vi "KIMTest.vi"() -> ()   [LabVIEW 2018, in "KIM101lib.lvlib"]
doc: "Use this template to build a producer/consumer design pattern with events to produce queue items. Use this design pattern instead of the User Interface Event Handler pattern for user interfaces when you want to execute code asynchronously in response to an event without slowing the user interface responsiveness."
uses:
  KIM101lib.lvlib
panel:
  in  "APTPZMotor":refnum<k7>(container)
  out "状态":i32[](array[numeric])
  in  "设置0位":bool
  in  "轴4":T1
  in  "轴3":T2
  in  "轴2":T3
  in  "轴1":T3
  out "Position":i32[](array[numeric])
  in  "stop":bool
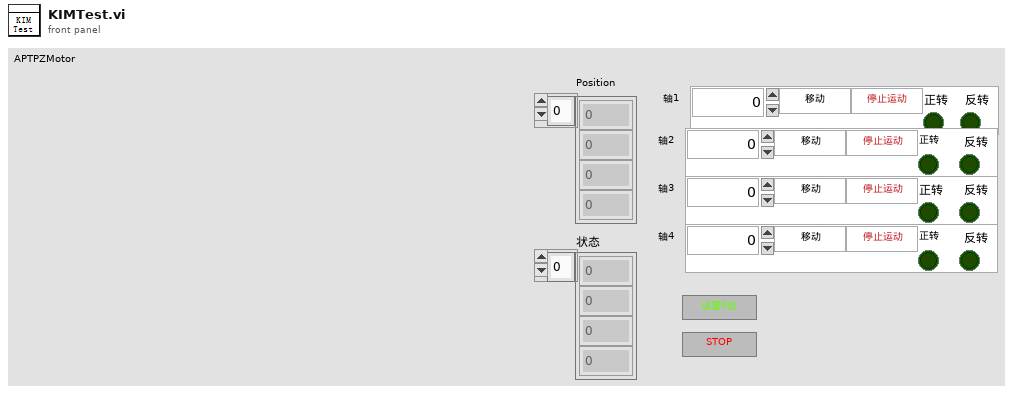
[diagram p1: front panel]
types:
  T1 = cluster{"目标位置":i32, "移动":bool, "停止运动":bool, "正转":bool, " 反转":bool}
  T2 = cluster{"目标位置":i32, "移动":bool, "停止运动":bool, "正转  ":bool, " 反转":bool}
  T3 = cluster{"目标位置":i32, "移动":bool, "停止运动":bool, "正转 ":bool, " 反转":bool}
  T4 = cluster{"电压(80-130)":i32, "速度(1-2000) ":i32, "加速度(1-100000)":i32}
  T5 = enum16{"全部禁用", "CH1使能", "CH2使能", "CH3使能", "CH4使能", "CH1,CH2使能", "CH3,CH4使能"}
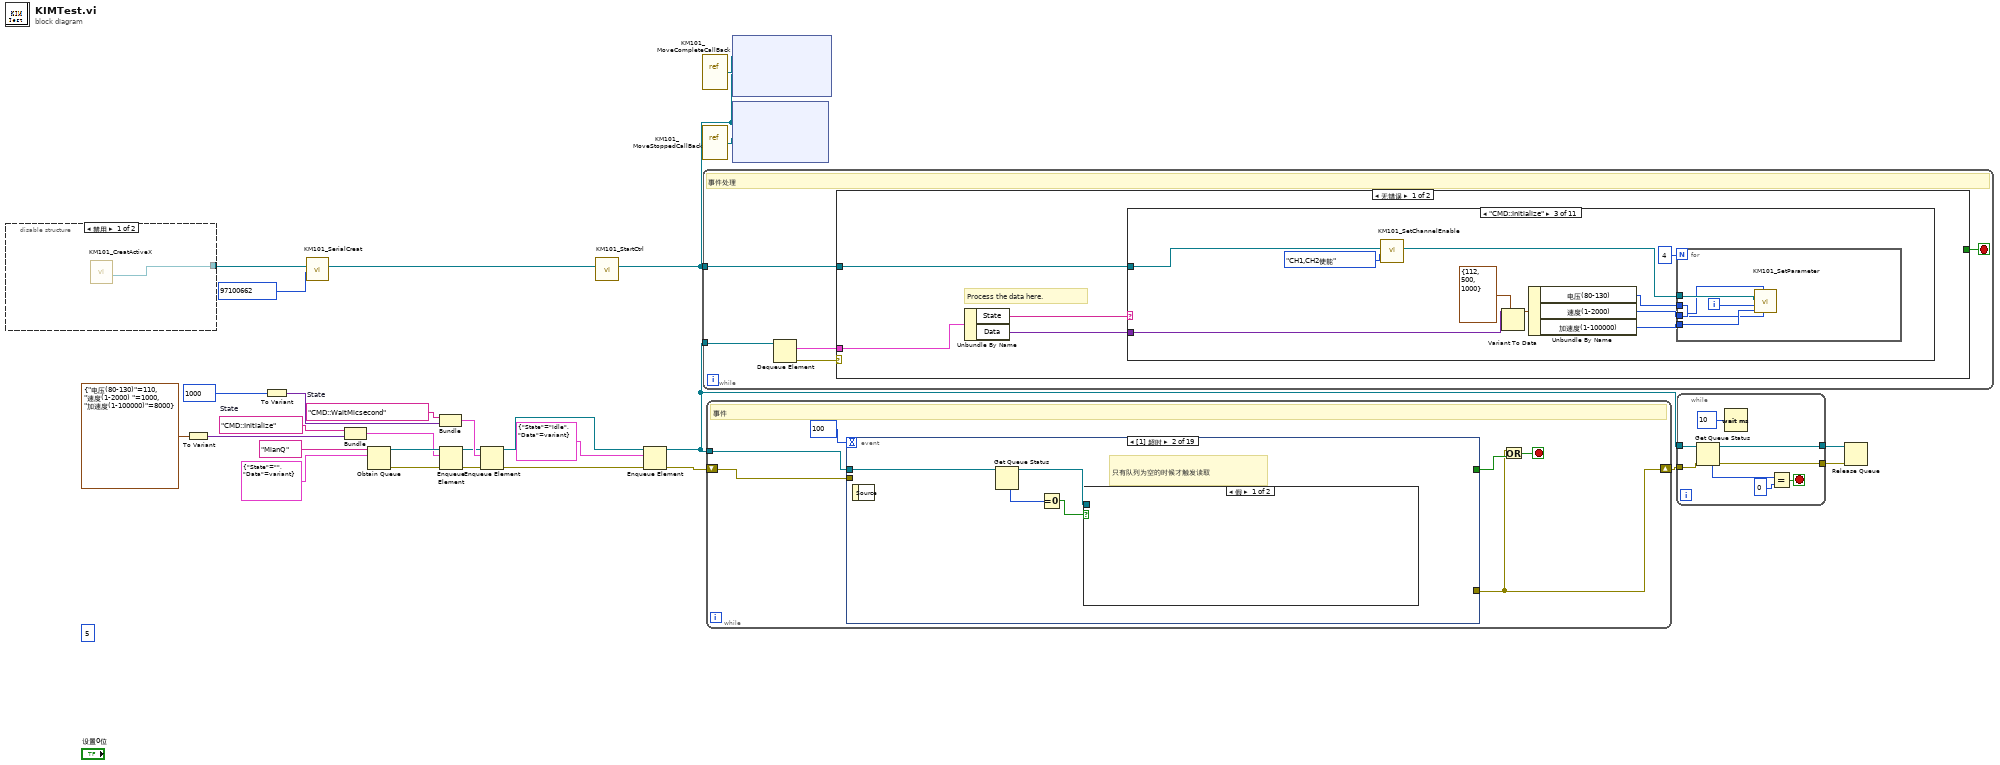
[diagram p0: block diagram]
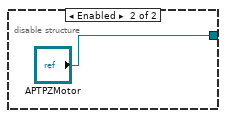
[diagram p2: hidden frame]
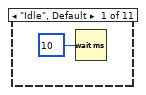
[diagram p3: hidden frame]
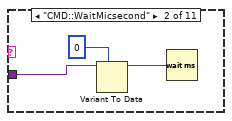
[diagram p4: hidden frame]
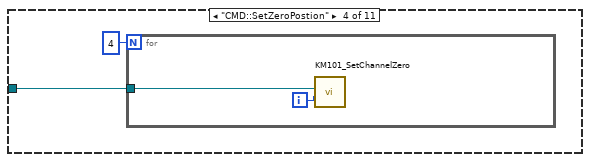
[diagram p5: hidden frame]
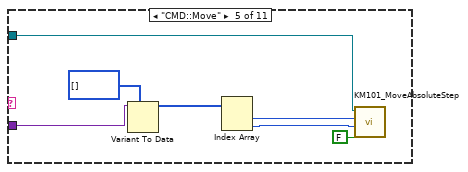
[diagram p6: hidden frame]
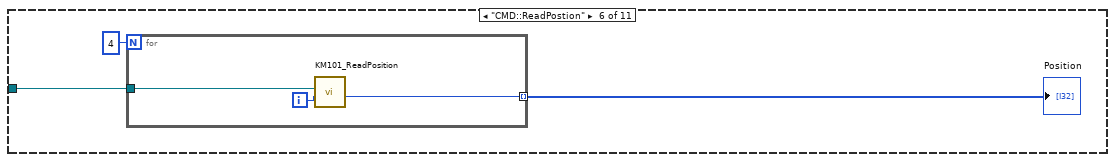
[diagram p7: hidden frame]
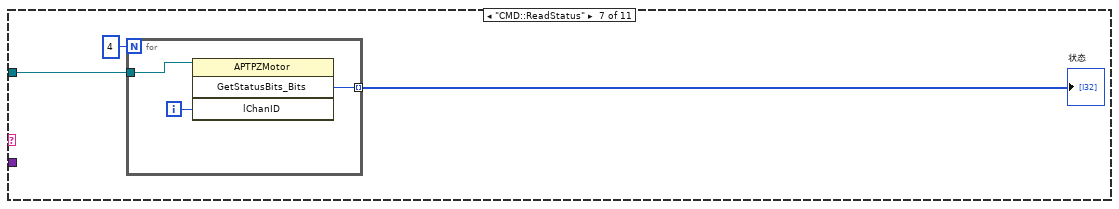
[diagram p8: hidden frame]
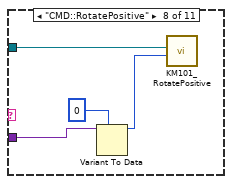
[diagram p9: hidden frame]
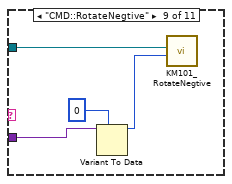
[diagram p10: hidden frame]
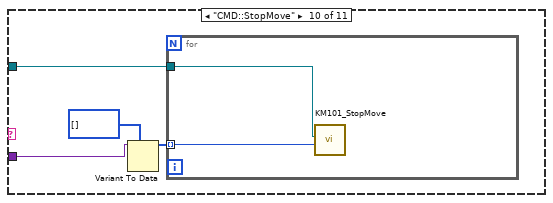
[diagram p11: hidden frame]
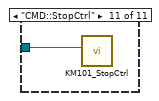
[diagram p12: hidden frame]
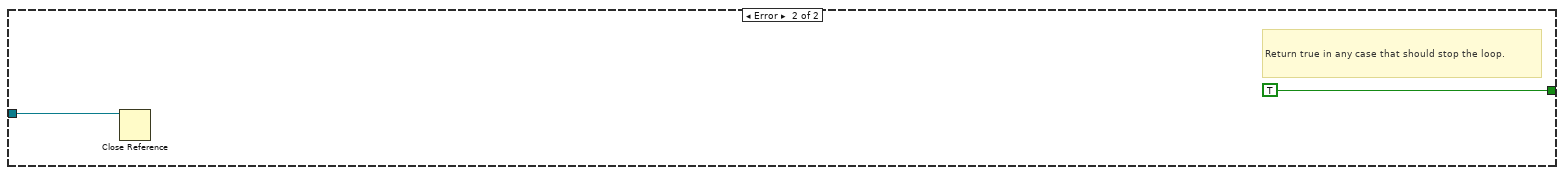
[diagram p13: hidden frame]
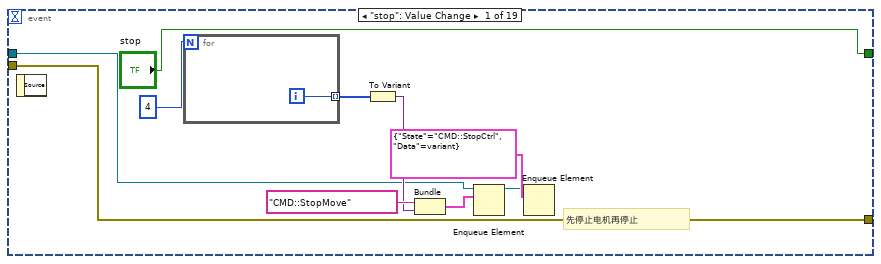
[diagram p14: hidden frame]
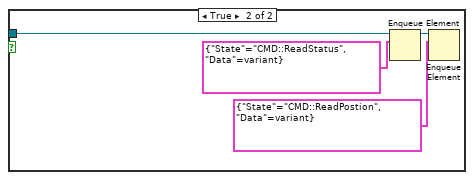
[diagram p15: hidden frame]
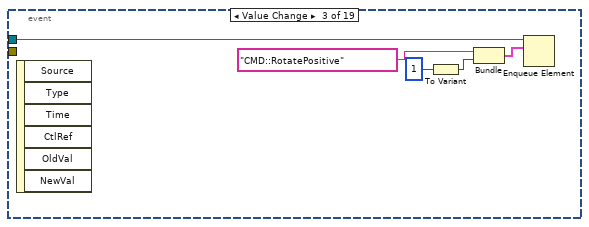
[diagram p16: hidden frame]
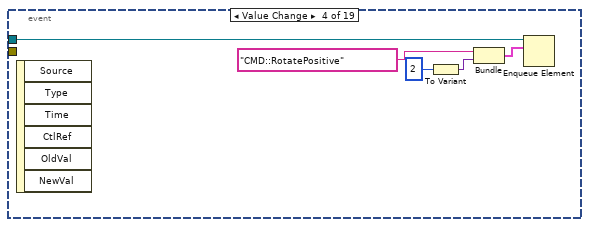
[diagram p17: hidden frame]
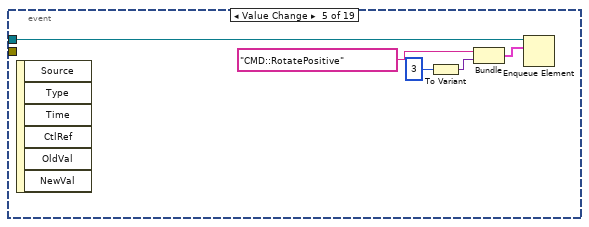
[diagram p18: hidden frame]
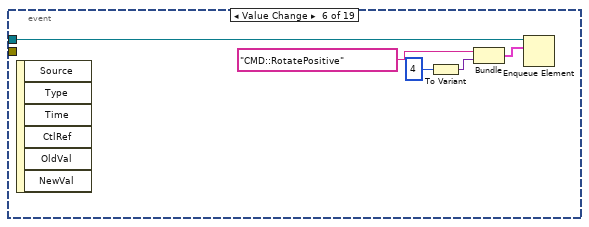
[diagram p19: hidden frame]
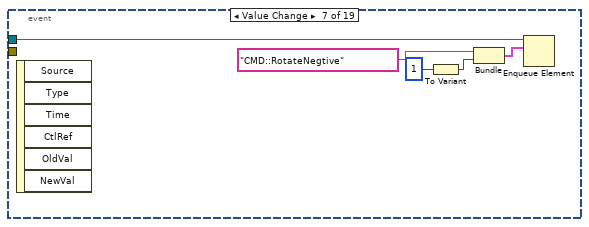
[diagram p20: hidden frame]
diagram:
  (unwired) 5 ("lMode")
  w9 = "CMD::Initialize"  # State
  w18 = "CMD::WaitMicsecond"  # State
  n1 = disable-structure shown="禁用" {
    disable-tunnel: [w29 "APTPZMotor"] -> w1
    frame Disabled {
      n2 = call "KM101_CreatActiveX.vi"() -> ("KIM引用"=w29:refnum<k7>)  [unwired: 11 in]
    }
    frame Enabled {
    }
  }
  n3 = To Variant(anything=T4 {"电压(80-130)"=110, "速度(1-2000) "=1000, "加速度(1-100000)"=8000}) -> (Variant=w7:variant)
  n4 = To Variant(anything=1000) -> (Variant=w17:variant)
  n5 = call "KM101_SerialCreat.vi"("HWSerialNum"=97100662, "reference in"=w1) -> ("reference out"=w2:refnum<k7>)  [unwired: 9 in]
  n6 = Bundle("State"=w9, "Variant"=w7) -> (w6:cluster{"State":string, "Variant":variant})  [unwired: 1 in]
  n7 = Obtain Queue(name (unnamed)="MianQ", element data type=cluster{"State":string, "Data":variant} {"State"="", "Data"=variant}) -> (queue out=w26:refnum<queue>, error out=w24:errorcluster)  [unwired: 3 in, 1 out]
  n8 = Bundle("State"=w18, "Variant"=w17) -> (w16:cluster{"State":string, "Variant":variant})  [unwired: 1 in]
  n9 = Enqueue Element(queue=w26, element=w6, error in (no error)=w24) -> (queue out=w15:refnum<queue>, error out=w13:errorcluster)  [unwired: 1 in, 1 out]
  n10 = Enqueue Element(queue=w15, element=w16, error in (no error)=w13) -> (queue out=w14:refnum<queue>, error out=w12:errorcluster)  [unwired: 1 in, 1 out]
  n11 = call "KM101_StartCtrl.vi"("reference in"=w2) -> ("reference out"=w3:refnum<k7>)  [unwired: 10 in]
  n12 = Enqueue Element(queue=w14, element=cluster{"State":string, "Data":variant} {"State"="Idle", "Data"=variant}, error in (no error)=w12) -> (queue out=w25:refnum<queue>, error out=w10:errorcluster)  [unwired: 1 in, 1 out]
  n13 = vi-ref "KM101_MoveCompleteCallBack.vi"() -> ("vi reference"=w5:refnum<vi>)
  n14 = vi-ref "KM101_MoveStoppedCallBack.vi"() -> (w4:refnum<vi>)
  n15 = while {
    tunnel: w25 -> [w35]
    tunnel: w3 -> [w31]
    stop <- w32 stop-if-true
    # "事件处理"
    n16 = Dequeue Element(queue=w35) -> (element=w33:cluster{"State":string, "Data":variant}, error out=w34:errorcluster)  [unwired: 2 in, 2 out]
    n17 = case shown="无错误" w34 {
      tunnel: w33 -> [w39 _]
      tunnel: [_ TRUE] -> w32
      tunnel: w31 -> [w37 w97]
      frame No Error {
        # "Process the data here."
        n18 = Unbundle By Name(w39) -> ("State"=w38:string, "Data"=w36:variant)
        n19 = case shown="\"CMD::Initialize\"" w38 {
          tunnel: w37 -> [_ _ w46 w60 w66 w72 w78 w85 w87 w90 w96]
          tunnel: w36 -> [_ w42 w52 _ w69 _ _ w84 w86 w92 _]
          frame "Idle", Default {
            n20 = Wait (ms)(milliseconds to wait=u32 10) -> ()  [unwired: 1 out]
          }
          frame "CMD::WaitMicsecond" {
            n21 = Variant To Data(type=u32 0 ("milliseconds to wait"), Variant=w42) -> (data=w41:u32)  [unwired: 1 in, 1 out]
            n22 = Wait (ms)(milliseconds to wait=w41) -> ()  [unwired: 1 out]
          }
          frame "CMD::Initialize" {
            n23 = call "KM101_SetChannelEnable.vi"("使能模式"=T5."CH1,CH2使能", "reference in"=w46) -> ("reference out"=w45:refnum<k7>)  [unwired: 9 in]
            n24 = Variant To Data(type=T4 {"电压(80-130)"=112, "速度(1-2000) "=500, "加速度(1-100000)"=1000}, Variant=w52) -> (data=w50:T4)  [unwired: 1 in, 1 out]
            n25 = Unbundle By Name(w50) -> ("电压(80-130)"=w49:i32, "速度(1-2000)"=w48:i32, "加速度(1-100000)"=w47:i32)
            n26 = for {
              N: 4 -> [_]
              tunnel: w45 -> [w58]
              tunnel: w49 -> [w54]
              tunnel: w48 -> [w55]
              tunnel: w47 -> [w56]
              i -> [w57]
              n27 = call "KM101_SetParameter.vi"("lVoltage"=w54, "lStepRate"=w55, "lStepAccn"=w56, "Channel"=w57, "reference in"=w58) -> ()  [unwired: 6 in, 1 out]
            }
          }
          frame "CMD::SetZeroPostion" {
            n28 = for {
              N: 4 -> [_]
              tunnel: w60 -> [w62]
              i -> [w61]
              n29 = call "KM101_SetChannelZero.vi"("Channel"=w61, "reference in"=w62) -> ()  [unwired: 9 in, 1 out]
            }
          }
          frame "CMD::Move" {
            n30 = Variant To Data(type=i32[] [], Variant=w69) -> (data=w67:i32[])  [unwired: 1 in, 1 out]
            n31 = Index Array(array=w67) -> (element #1=w65:i32, element #2=w64:i32)  [unwired: 2 in]
            n32 = call "KM101_MoveAbsoluteStep.vi"("bWait"=FALSE, "AbsSteps"=w64, "Channel"=w65, "reference in"=w66) -> ()  [unwired: 7 in, 1 out]
          }
          frame "CMD::ReadPostion" {
            n33 = for {
              N: 4 -> [_]
              tunnel: w72 -> [w75]
              tunnel: [w73] -> w70 mode=indexing
              i -> [w74]
              n34 = call "KM101_ReadPosition.vi"("Channel"=w74, "reference in"=w75) -> ("Steps"=w73:i32)  [unwired: 8 in, 1 out]
            }
            "Position" <- w70
          }
          frame "CMD::ReadStatus" {
            n35 = for {
              N: 4 -> [_]
              tunnel: w78 -> [w81]
              tunnel: [w79] -> w76 mode=indexing
              i -> [w80]
              n36 = invoke class="APTPZMotor" method="GetStatusBits_Bits"(reference=w81, "lChanID"=w80) -> ("GetStatusBits_Bits"=w79:i32)  [unwired: 2 in, 3 out]
            }
            "状态" <- w76
          }
          frame "CMD::RotatePositive" {
            n37 = Variant To Data(type=0, Variant=w84) -> (data=w82:i32)  [unwired: 1 in, 1 out]
            n38 = call "KM101_RotatePositive.vi"("Channel"=w82, "reference in"=w85) -> ()  [unwired: 8 in, 2 out]
          }
          frame "CMD::RotateNegtive" {
            n39 = Variant To Data(type=0, Variant=w86) -> (data=w88:i32)  [unwired: 1 in, 1 out]
            n40 = call "KM101_RotateNegtive.vi"("Channel"=w88, "reference in"=w87) -> ()  [unwired: 8 in, 2 out]
          }
          frame "CMD::StopMove" {
            n41 = Variant To Data(type=i32[] [], Variant=w92) -> (data=w91:i32[])  [unwired: 1 in, 1 out]
            n42 = for {
              tunnel: w91 -> [w94] mode=indexing
              tunnel: w90 -> [w95]
              n43 = call "KM101_StopMove.vi"("Channel"=w94, "reference in"=w95) -> ()  [unwired: 9 in, 1 out]
            }
          }
          frame "CMD::StopCtrl" {
            n44 = call "KM101_StopCtrl.vi"("reference in"=w96) -> ()  [unwired: 11 in]
          }
        }
      }
      frame Error {
        # "Return true in any case that should stop the loop."
        n45 = Close Reference(reference=w97) -> ()  [unwired: 1 in, 1 out]
      }
    }
  }
  n46 = while {
    shift-right: [w100] -> w21
    shift-left: w10 -> [w103]
    tunnel: w25 -> [w104]
    stop <- w101 stop-if-true
    # "事件"
    n47 = event shown="[1] 超时" {
      selector: _ -> [_ _ _ _ _ _ _ _ _ _ _ _ _ _ _ _ _ _ _]
      dyn-events: _ -> [_ _ _ _ _ _ _ _ _ _ _ _ _ _ _ _ _ _ _]
      timeout: 100 -> [_ _ _ _ _ _ _ _ _ _ _ _ _ _ _ _ _ _ _]
      tunnel: w104 -> [w105 w119 w124 w129 w134 w139 w144 w149 w154 w159 w164 w173 w183 w193 w202 w207 w215 w223 w231]
      tunnel: w103 -> [w113 _ _ _ _ _ _ _ _ _ _ _ _ _ _ _ _ _ _]
      tunnel: [w113 _ _ _ _ _ _ _ _ _ _ _ _ _ _ _ _ _ _] -> w100
      tunnel: ["stop" _ _ _ _ _ _ _ _ _ _ _ _ _ _ _ _ _ _] -> w102
      event "stop": Value Change {
        # "先停止电机再停止"
        n48 = event-data() -> ()  [unwired: 1 in, 1 out]
        n49 = for {
          N: 4 -> [_]
          tunnel: [w115] -> w111 mode=indexing
          i -> [w115]
        }
        n50 = To Variant(anything=w111) -> (Variant=w109:variant)
        n51 = Bundle("State"="CMD::StopMove", "Variant"=w109) -> (w108:cluster{"State":string, "Variant":variant})  [unwired: 1 in]
        n52 = Enqueue Element(queue=w105, element=w108) -> (queue out=w107:refnum<queue>)  [unwired: 2 in, 2 out]
        n53 = Enqueue Element(queue=w107, element=cluster{"State":string, "Data":variant} {"State"="CMD::StopCtrl", "Data"=variant}) -> ()  [unwired: 2 in, 3 out]
      }
      event Timeout {
        # "只有队列为空的时候才触发读取"
        n54 = event-data() -> ()  [unwired: 1 in, 1 out]
        n55 = Get Queue Status(queue=w119) -> (queue out=w116:refnum<queue>, # elements in queue=w118:i32)  [unwired: 2 in, 6 out]
        n56 = Equal To 0?(x=w118) -> (x = 0?=w117:bool)
        n57 = case shown="假" w117 {
          tunnel: w116 -> [_ w122]
          frame False {
          }
          frame True {
            n58 = Enqueue Element(queue=w122, element=cluster{"State":string, "Data":variant} {"State"="CMD::ReadStatus", "Data"=variant}) -> (queue out=w121:refnum<queue>)  [unwired: 2 in, 2 out]
            n59 = Enqueue Element(queue=w121, element=cluster{"State":string, "Data":variant} {"State"="CMD::ReadPostion", "Data"=variant}) -> ()  [unwired: 2 in, 3 out]
          }
        }
      }
      event "轴1.正转": Value Change {
        n60 = event-data() -> ()  [unwired: 1 in, 6 out]
        n61 = To Variant(anything=1) -> (Variant=w127:variant)
        n62 = Bundle("State"="CMD::RotatePositive", "Variant"=w127) -> (w125:cluster{"State":string, "Variant":variant})  [unwired: 1 in]
        n63 = Enqueue Element(queue=w124, element=w125) -> ()  [unwired: 2 in, 3 out]
      }
      event "轴2.正转": Value Change {
        n64 = event-data() -> ()  [unwired: 1 in, 6 out]
        n65 = To Variant(anything=2) -> (Variant=w132:variant)
        n66 = Bundle("State"="CMD::RotatePositive", "Variant"=w132) -> (w130:cluster{"State":string, "Variant":variant})  [unwired: 1 in]
        n67 = Enqueue Element(queue=w129, element=w130) -> ()  [unwired: 2 in, 3 out]
      }
      event "轴3.正转": Value Change {
        n68 = event-data() -> ()  [unwired: 1 in, 6 out]
        n69 = To Variant(anything=3) -> (Variant=w137:variant)
        n70 = Bundle("State"="CMD::RotatePositive", "Variant"=w137) -> (w135:cluster{"State":string, "Variant":variant})  [unwired: 1 in]
        n71 = Enqueue Element(queue=w134, element=w135) -> ()  [unwired: 2 in, 3 out]
      }
      event "轴4.正转": Value Change {
        n72 = event-data() -> ()  [unwired: 1 in, 6 out]
        n73 = To Variant(anything=4) -> (Variant=w142:variant)
        n74 = Bundle("State"="CMD::RotatePositive", "Variant"=w142) -> (w140:cluster{"State":string, "Variant":variant})  [unwired: 1 in]
        n75 = Enqueue Element(queue=w139, element=w140) -> ()  [unwired: 2 in, 3 out]
      }
      event "轴1.反转": Value Change {
        n76 = event-data() -> ()  [unwired: 1 in, 6 out]
        n77 = To Variant(anything=1) -> (Variant=w147:variant)
        n78 = Bundle("State"="CMD::RotateNegtive", "Variant"=w147) -> (w145:cluster{"State":string, "Variant":variant})  [unwired: 1 in]
        n79 = Enqueue Element(queue=w144, element=w145) -> ()  [unwired: 2 in, 3 out]
      }
      event "轴2.反转": Value Change {
        n80 = event-data() -> ()  [unwired: 1 in, 6 out]
        n81 = To Variant(anything=2) -> (Variant=w152:variant)
        n82 = Bundle("State"="CMD::RotateNegtive", "Variant"=w152) -> (w150:cluster{"State":string, "Variant":variant})  [unwired: 1 in]
        n83 = Enqueue Element(queue=w149, element=w150) -> ()  [unwired: 2 in, 3 out]
      }
      event "轴3.反转": Value Change {
        n84 = event-data() -> ()  [unwired: 1 in, 6 out]
        n85 = To Variant(anything=3) -> (Variant=w157:variant)
        n86 = Bundle("State"="CMD::RotateNegtive", "Variant"=w157) -> (w155:cluster{"State":string, "Variant":variant})  [unwired: 1 in]
        n87 = Enqueue Element(queue=w154, element=w155) -> ()  [unwired: 2 in, 3 out]
      }
      event "轴4.反转": Value Change {
        n88 = event-data() -> ()  [unwired: 1 in, 6 out]
        n89 = To Variant(anything=4) -> (Variant=w162:variant)
        n90 = Bundle("State"="CMD::RotateNegtive", "Variant"=w162) -> (w160:cluster{"State":string, "Variant":variant})  [unwired: 1 in]
        n91 = Enqueue Element(queue=w159, element=w160) -> ()  [unwired: 2 in, 3 out]
      }
      event "设置0位": Value Change {
        n92 = event-data() -> ()  [unwired: 1 in, 6 out]
        n93 = Enqueue Element(queue=w164, element=cluster{"State":string, "Data":variant} {"State"="CMD::SetZeroPostion", "Data"=variant}) -> ()  [unwired: 2 in, 3 out]
      }
      event "轴1.移动": Value Change {
        w176 = "CMD::Move"  # State
        n94 = event-data() -> ("CtlRef"=w168:refnum<vi>, "NewVal"=w167:bool)  [unwired: 1 in]
        n95 = Unbundle By Name("轴1") -> ("目标位置"=w170:i32)
        n96 = Not(x=w167) -> (.not. x?=w166:bool)
        n97 = call "KeyGray.vi"("Value"=w166, "CtlRef"=w168) -> ()  [unwired: 10 in]
        n98 = Build Array(0, w170) -> (w169:i32[])
        n99 = To Variant(anything=w169) -> (Variant=w175:variant)
        n100 = Bundle("State"=w176, "Variant"=w175) -> (w172:cluster{"State":string, "Variant":variant})  [unwired: 1 in]
        n101 = Enqueue Element(queue=w173, element=w172) -> ()  [unwired: 2 in, 3 out]
      }
      event "轴2.移动": Value Change {
        w186 = "CMD::Move"  # State
        n102 = event-data() -> ("CtlRef"=w178:refnum<vi>, "OldVal"=w177:bool)  [unwired: 1 in]
        n103 = call "KeyGray.vi"("Value"=w177, "CtlRef"=w178) -> ()  [unwired: 10 in]
        n104 = Unbundle By Name("轴2") -> ("目标位置"=w181:i32)
        n105 = Build Array(1, w181) -> (w179:i32[])
        n106 = To Variant(anything=w179) -> (Variant=w185:variant)
        n107 = Bundle("State"=w186, "Variant"=w185) -> (w184:cluster{"State":string, "Variant":variant})  [unwired: 1 in]
        n108 = Enqueue Element(queue=w183, element=w184) -> ()  [unwired: 2 in, 3 out]
      }
      event "轴3.移动": Value Change {
        w195 = "CMD::Move"  # State
        n109 = event-data() -> ("CtlRef"=w188:refnum<vi>, "OldVal"=w187:bool)  [unwired: 1 in]
        n110 = call "KeyGray.vi"("Value"=w187, "CtlRef"=w188) -> ()  [unwired: 10 in]
        n111 = Unbundle By Name("轴3") -> ("目标位置"=w191:i32)
        n112 = Build Array(2, w191) -> (w190:i32[])
        n113 = Bundle("State"=w195, w190) -> (w194:cluster{"State":string, i32[]})  [unwired: 1 in]
        n114 = Enqueue Element(queue=w193, element=w194) -> ()  [unwired: 2 in, 3 out]
      }
      event "轴4.移动": Value Change {
        w204 = "CMD::Move"  # State
        n115 = event-data() -> ("CtlRef"=w197:refnum<vi>, "OldVal"=w196:bool)  [unwired: 1 in]
        n116 = call "KeyGray.vi"("Value"=w196, "CtlRef"=w197) -> ()  [unwired: 10 in]
        n117 = Unbundle By Name("轴4") -> ("目标位置"=w200:i32)
        n118 = Build Array(3, w200) -> (w199:i32[])
        n119 = Bundle("State"=w204, w199) -> (w203:cluster{"State":string, i32[]})  [unwired: 1 in]
        n120 = Enqueue Element(queue=w202, element=w203) -> ()  [unwired: 2 in, 3 out]
      }
      event "轴1.停止运动": Value Change {
        w212 = "CMD::StopMove"  # State
        n121 = event-data() -> ("CtlRef"=w206:refnum<vi>, "OldVal"=w205:bool)  [unwired: 1 in]
        n122 = call "KeyGray.vi"("Value"=w205, "CtlRef"=w206) -> ()  [unwired: 10 in]
        n123 = Build Array(0) -> (w209:i32[])
        n124 = To Variant(anything=w209) -> (Variant=w211:variant)
        n125 = Bundle("State"=w212, "Variant"=w211) -> (w208:cluster{"State":string, "Variant":variant})  [unwired: 1 in]
        n126 = Enqueue Element(queue=w207, element=w208) -> ()  [unwired: 2 in, 3 out]
      }
      event "轴2.停止运动": Value Change {
        w220 = "CMD::StopMove"  # State
        n127 = event-data() -> ("CtlRef"=w214:refnum<vi>, "OldVal"=w213:bool)  [unwired: 1 in]
        n128 = call "KeyGray.vi"("Value"=w213, "CtlRef"=w214) -> ()  [unwired: 10 in]
        n129 = Build Array(1) -> (w217:i32[])
        n130 = To Variant(anything=w217) -> (Variant=w219:variant)
        n131 = Bundle("State"=w220, "Variant"=w219) -> (w216:cluster{"State":string, "Variant":variant})  [unwired: 1 in]
        n132 = Enqueue Element(queue=w215, element=w216) -> ()  [unwired: 2 in, 3 out]
      }
      event "轴3.停止运动": Value Change {
        w228 = "CMD::StopMove"  # State
        n133 = event-data() -> ("CtlRef"=w222:refnum<vi>, "OldVal"=w221:bool)  [unwired: 1 in]
        n134 = call "KeyGray.vi"("Value"=w221, "CtlRef"=w222) -> ()  [unwired: 10 in]
        n135 = Build Array(2) -> (w225:i32[])
        n136 = To Variant(anything=w225) -> (Variant=w227:variant)
        n137 = Bundle("State"=w228, "Variant"=w227) -> (w224:cluster{"State":string, "Variant":variant})  [unwired: 1 in]
        n138 = Enqueue Element(queue=w223, element=w224) -> ()  [unwired: 2 in, 3 out]
      }
      event "轴4.停止运动": Value Change {
        w236 = "CMD::StopMove"  # State
        n139 = event-data() -> ("CtlRef"=w230:refnum<vi>, "OldVal"=w229:bool)  [unwired: 1 in]
        n140 = call "KeyGray.vi"("Value"=w229, "CtlRef"=w230) -> ()  [unwired: 10 in]
        n141 = Build Array(3) -> (w233:i32[])
        n142 = To Variant(anything=w233) -> (Variant=w235:variant)
        n143 = Bundle("State"=w236, "Variant"=w235) -> (w232:cluster{"State":string, "Variant":variant})  [unwired: 1 in]
        n144 = Enqueue Element(queue=w231, element=w232) -> ()  [unwired: 2 in, 3 out]
      }
    }
    n145 = Or(x=w100, y=w102) -> (x .or. y?=w101:bool)
  }
  n146 = node(w3, w5) -> ()  [unwired: 3 in, 2 out]
  n147 = node(w3, w4) -> ()  [unwired: 3 in, 2 out]
  n148 = while {
    tunnel: w25 -> [w244]
    tunnel: [w243] -> w22
    tunnel: w21 -> [w242]
    tunnel: [w241] -> w20
    stop <- w238 stop-if-true
    n149 = Get Queue Status(queue=w244, error in (no error)=w242) -> (queue out=w243:refnum<queue>, error out=w241:errorcluster, # elements in queue=w240:i32)  [unwired: 1 in, 5 out]
    n150 = Wait (ms)(milliseconds to wait=u32 10) -> ()  [unwired: 1 out]
    n151 = Equal?(x=w240, y=0) -> (x = y?=w238:bool)
  }
  n152 = Release Queue(queue=w22, error in (no error)=w20) -> ()  [unwired: 1 in, 3 out]
